vi "Prompt for Inverter Name.vi"(8 "error in (no error)":errorcluster, 9 "bypass (F)":bool, 10 "Name":string) -> (0 "error out":errorcluster, 1 "canceled":bool, 2 "name out":string)   [LabVIEW 2019, in "Main.lvclass"]
doc: "Developed by Kevin Thompson\nkevin@thompsonengineering.net\n\nCopyright 2020\nThompson Engineering, LLC"
uses:
  Main.lvclass
panel:
  in  "Cancel":bool
  in  "OK":bool
  # "Please Provide A Unique Name\nFor This Inverter"
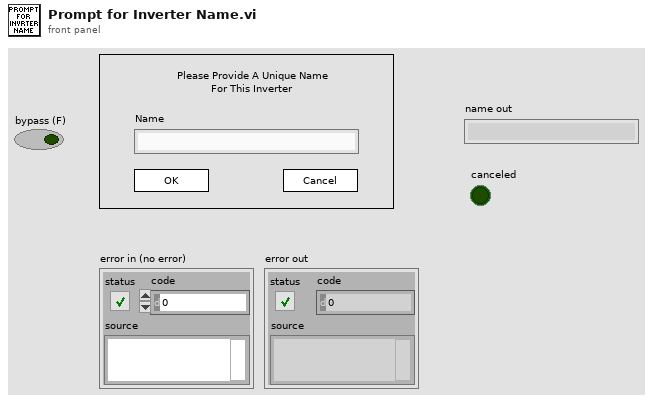
[diagram p1: front panel]
types:
  T1 = enum32{"Invalid", "Default", "Floating", "Floating/Auto-Hide", "Modal"}
  T2 = enum32{"Invalid", "Standard", "Closed", "Hidden", "Minimized", "Maximized"}
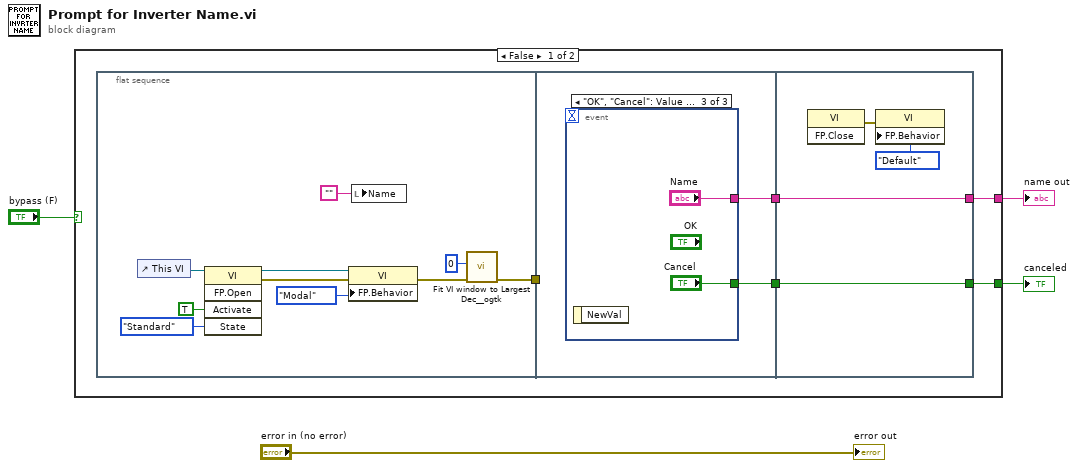
[diagram p0: block diagram]
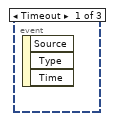
[diagram p2: hidden frame]
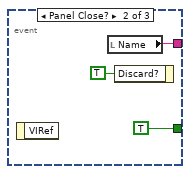
[diagram p3: hidden frame]
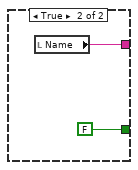
[diagram p4: hidden frame]
diagram:
  n1 = case shown="False" "bypass (F)" {
    tunnel: [w6 FALSE ("Cancel")] -> w3
    tunnel: [w5 w31] -> w2
    frame False {
      n2 = flat-sequence {
        tunnel: [w11] -> w9
        tunnel: [w21] -> w8
        tunnel: [w20] -> w7
        tunnel: w9 -> [_]
        tunnel: w8 -> [w27]
        tunnel: w7 -> [w28]
        tunnel: [w28] -> w6
        tunnel: [w27] -> w5
        frame #0 {
          n3 = control-ref of="This VI"() -> (w12:refnum<vi>)
          n4 = invoke class="VI" method="FP.Open"(reference=w12, "Activate"=TRUE ("Activate?"), "State"=T2."Standard") -> (reference out=w19:refnum<vi>, error out=w17:errorcluster)  [unwired: 2 in, 3 out]
          n5 = property class="VI"(reference=w19, error in=w17, "FP.Behavior"=T1."Modal" ("Front Panel Window:Behavior")) -> (error out=w18:errorcluster)  [unwired: 1 out]
          n6 = local write "Name"("") -> ()
          n7 = call <userlib>:"Fit VI window to Largest Dec__ogtk.vi"("error in (no error)"=w18, "border spacing (2 px)"=0) -> ("error out"=w11:errorcluster)  [unwired: 4 in, 1 out]
        }
        frame #1 {
          n8 = event shown="[2] \"OK\", \"Cancel\": Value Change" {
            selector: _ -> [_ _ _]
            dyn-events: _ -> [_ _ _]
            timeout: _ -> [_ _ _]
            tunnel: [_ w23 "Name"] -> w21
            tunnel: [_ TRUE ("Cancel") "Cancel"] -> w20
            event Timeout {
              n9 = event-data() -> ()  [unwired: 1 in, 3 out]
            }
            event Panel Close? {
              n10 = event-data() -> ()  [unwired: 1 in, 1 out]
              n11 = local read "Name"() -> (w23:string)
              n12 = event-data("Discard?"=TRUE) -> ()  [unwired: 1 in, 1 out]
            }
            event "OK", "Cancel": Value Change {
              n13 = event-data() -> ()  [unwired: 1 in, 1 out]
            }
          }
        }
        frame #2 {
          n14 = invoke class="VI" method="FP.Close"() -> (error out=w30:errorcluster)  [unwired: 3 in, 2 out]
          n15 = property class="VI"(error in=w30, "FP.Behavior"=T1."Default" ("Front Panel Window:Behavior")) -> ()  [unwired: 1 in, 2 out]
        }
      }
    }
    frame True {
      n16 = local read "Name"() -> (w31:string)
    }
  }
  "canceled" <- w3
  "name out" <- w2
  "error out" <- "error in (no error)"
